vi "DistanceToTargetMath.vi"(2 "TargetCenter":dbl) -> (0 "DistancetoTarget":dbl)   [LabVIEW 2016]
panel:
  in  "CameraAngleofElevation":dbl=44.285
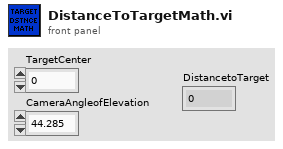
[diagram p1: front panel]
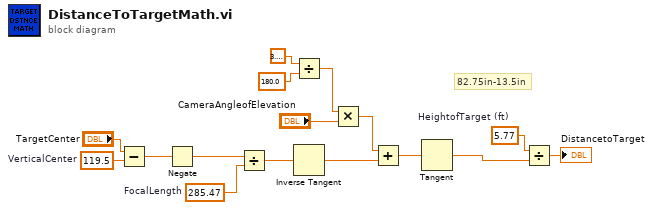
[diagram p0: block diagram]
diagram:
  w3 = 119.5  # VerticalCenter
  w13 = 285.47  # FocalLength
  w16 = 5.77  # HeightofTarget (ft)
  # "82.75in-13.5in"
  n1 = Subtract(x="TargetCenter", y=w3) -> (x-y=w2:dbl)
  n2 = Negate(x=w2) -> (-x=w1:dbl)
  n3 = Divide(x=w1, y=w13) -> (x/y=w14:dbl)
  n4 = Divide(x=3.141592653589793, y=180.0 ("x")) -> (x/y=w6:dbl)
  n5 = Inverse Tangent(1:w14) -> (0:w8:dbl)
  n6 = Multiply(x=w6, y="CameraAngleofElevation") -> (x*y=w5:dbl)
  n7 = Add(x=w5, y=w8) -> (x+y=w15:dbl)
  n8 = Tangent(1:w15) -> (0:w11:dbl)
  n9 = Divide(x=w16, y=w11) -> (x/y=→"DistancetoTarget":dbl)
